vi "Pre Launch Init.vi"(11 "Chamber Pressure in":refnum<class "Chamber Pressure.lvclass">) -> (0 "error out":errorcluster, 3 "Chamber Pressure out":refnum<class "Chamber Pressure.lvclass">)   [LabVIEW 2018, in "Pressure Actor.lvlib" / "Chamber Pressure.lvclass"]
doc: "(<B>Filename</B>: Actor Framework.lvlib:Actor.lvclass:Pre Launch Init.vi)\n\nDefines behavior that occurs after the Launch Nested Actor method is invoked but before the actor's Actor Core method begins running.\n\nBy default, this method does nothing. A descendant class may override it to define behavior."
uses:
  Chamber Pressure.lvclass
  Chamber Pressure.lvclass/Chamber Pressure.ctl
  <vilib>/DAQmx/create/channels.llb/DAQmx Create Channel (AI-Voltage-Basic).vi
  Pressure/Pressure.lvclass
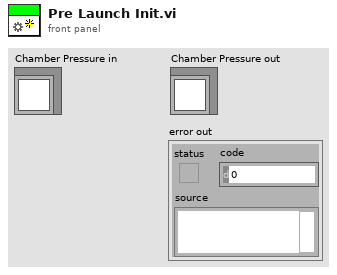
[diagram p1: front panel]
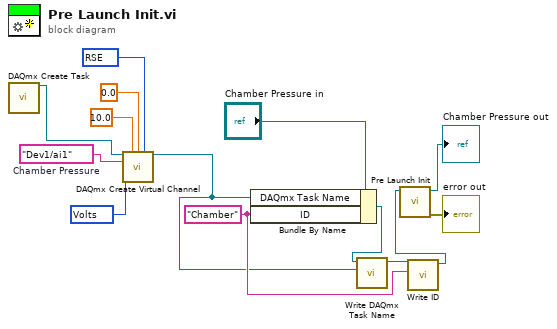
[diagram p0: block diagram]
diagram:
  w7 = 10083 items=["Default"=-1, "RSE"=10083, "NRSE"=10078, "Differential"=10106, "Pseudodifferential"=12529] ("input terminal configuration")
  w8 = 10348 items=["Volts"=10348, "From Custom Scale"=10065] ("units")
  w11 = tag "Dev1/ai1"  # Chamber Pressure
  w2 = "Chamber" ("ID")
  n1 = call <vilib>:"DAQmx Create Task.vi"() -> ("task out"=w6:refnum<k21>)  [unwired: 14 in, 1 out]
  n2 = call-poly <vilib>:"DAQmx Create Virtual Channel.vi"("task in"=w6, "maximum value"=10.0, "minimum value"=0.0, "input terminal configuration"=w7, "physical channels"=w11, "units"=w8) -> ("task out"=w1:refnum<k21>)  [unwired: 8 in, 1 out]
  n3 = Bundle By Name(cluster="Chamber Pressure in", "DAQmx Task Name"=w1, "ID"=w2) -> (w4:refnum<class "Chamber Pressure.lvclass">)
  n4 = call-dynamic "Write DAQmx Task Name.vi"("DAQmx Task Name"=w1, "Pressure in"=w4) -> ("Pressure out"=w5:refnum<class "Chamber Pressure.lvclass">)  [unwired: 8 in, 1 out]
  n5 = call-dynamic "Write ID.vi"("ID"=w2, "Pressure in"=w5) -> ("Pressure out"=w3:refnum<class "Chamber Pressure.lvclass">)  [unwired: 8 in, 1 out]
  n6 = call-parent "Pre Launch Init.vi"("Pressure in"=w3) -> ("error out"=→"error out":errorcluster, "Pressure out"=→"Chamber Pressure out":refnum<class "Chamber Pressure.lvclass">)  [unwired: 9 in]
